vi "6509_loop.vi"(8 "error in":errorcluster, 9 "read_spill_id":u32, 10 "file in":path, 11 "task":refnum<k21>) -> (0 "error out":errorcluster)   [LabVIEW 2018, in "6509.lvlib"]
uses:
  Libraries/6509/6509.lvlib
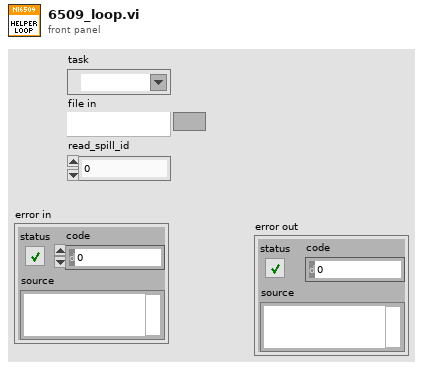
[diagram p1: front panel]
types:
  T1 = typedef "6509.lvlib/Request Events--cluster.ctl" = cluster{"Stop Module":refnum<user-event>, "Show Panel":refnum<user-event>, "Hide Panel":refnum<user-event>, "Get Module Execution Status":refnum<user-event>, "Show Diagram":refnum<user-event>, "Wakeup Helper Loop":refnum<user-event>, "Start Edge Detection":refnum<user-event>, "Stop Edge Detection":refnum<user-event>, "Pass Settings 4Helper":refnum<user-event>}
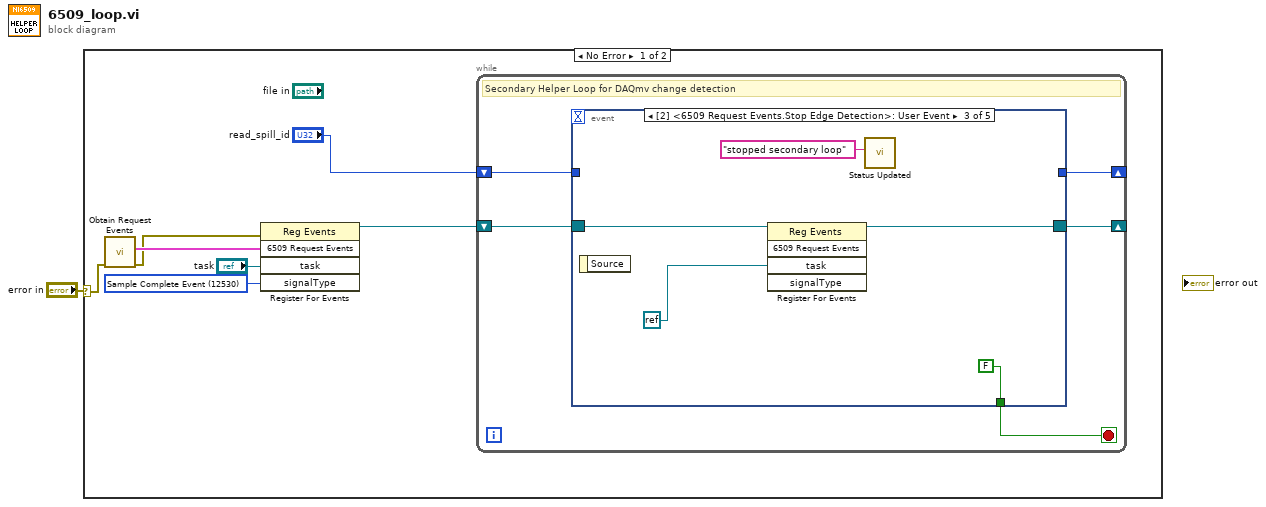
[diagram p0: block diagram]
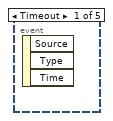
[diagram p2: hidden frame]
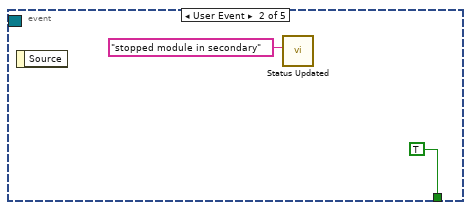
[diagram p3: hidden frame]
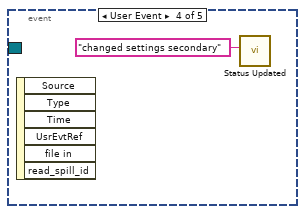
[diagram p4: hidden frame]
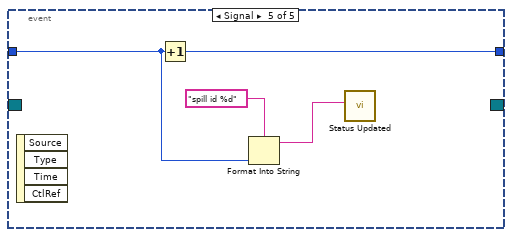
[diagram p5: hidden frame]
diagram:
  n1 = case shown="No Error" "error in" {
    selector: "error in" -> [w6 _]
    frame No Error {
      w3 = 12530 items=["Sample Complete Event"=12530, "Counter Output Event"=12494, "Change Detection Event"=12511, "Sample Clock"=12487] ("signalType")
      n2 = call "Obtain Request Events.vi"("error in (no error)"=w6) -> ("error out"=w5:errorcluster, "6509 Request Events"=w8:T1)  [unwired: 9 in]
      n3 = register-events(error in=w5, w8, "task", w3) -> (reference out=w7:refnum<event-registration>)  [unwired: 1 in, 1 out]
      n4 = while {
        shift-right: [w11] -> _
        shift-left: w7 -> [w13]
        shift-right: [w9] -> _
        shift-left: "read_spill_id" -> [w10]
        stop <- w12 stop-if-true
        # "Secondary Helper Loop for DAQmv change detection"
        n5 = event shown="[2] <6509 Request Events.Stop Edge Detection>: User Event" {
          selector: w13 -> [_ _ w18 _ _]
          dyn-events: [_ _ w16 _ _] -> w11
          timeout: _ -> [_ _ _ _ _]
          tunnel: [_ TRUE FALSE _ _] -> w12
          tunnel: w10 -> [_ _ _ _ w23]
          tunnel: [_ _ _ _ w25] -> w9
          event Timeout {
            n6 = event-data() -> ()  [unwired: 1 in, 3 out]
          }
          event User Event {
            n7 = event-data() -> ()  [unwired: 1 in, 1 out]
            n8 = call "Status Updated.vi"("Status"="stopped module in secondary") -> ()  [unwired: 10 in, 1 out]
          }
          event User Event {
            n9 = event-data() -> ()  [unwired: 1 in, 1 out]
            n10 = register-events(reference=w18, refnum<k0> refnum) -> (reference out=w16:refnum<event-registration>)  [unwired: 3 in, 1 out]
            n11 = call "Status Updated.vi"("Status"="stopped secondary loop") -> ()  [unwired: 10 in, 1 out]
          }
          event User Event {
            n12 = event-data() -> ()  [unwired: 1 in, 6 out]
            n13 = call "Status Updated.vi"("Status"="changed settings secondary") -> ()  [unwired: 10 in, 1 out]
          }
          event Signal {
            n14 = event-data() -> ()  [unwired: 1 in, 4 out]
            n15 = Increment(x=w23) -> (x+1=w25:u32)
            n16 = Format Into String(format string="spill id %d" ("Status"), w23) -> (resulting string=w22:string)  [unwired: 2 in, 1 out]
            n17 = call "Status Updated.vi"("Status"=w22) -> ()  [unwired: 10 in, 1 out]
          }
        }
      }
    }
    frame Error {
    }
  }
